vi "Get Enclosing Target Item.vi"(11 "tsRef":refnum<vi>) -> (3 "targetItem":refnum<vi>)   [LabVIEW 2020, in "NI_TargetHelper.lvlib"]
uses:
  <vilib>/TargetSupport/NI_TargetHelper/NI_TargetHelper.lvlib
  a0133eca-297a-364c-b9d3-27e53c6066f6.vi
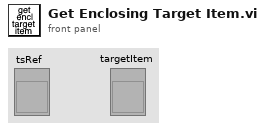
[diagram p1: front panel]
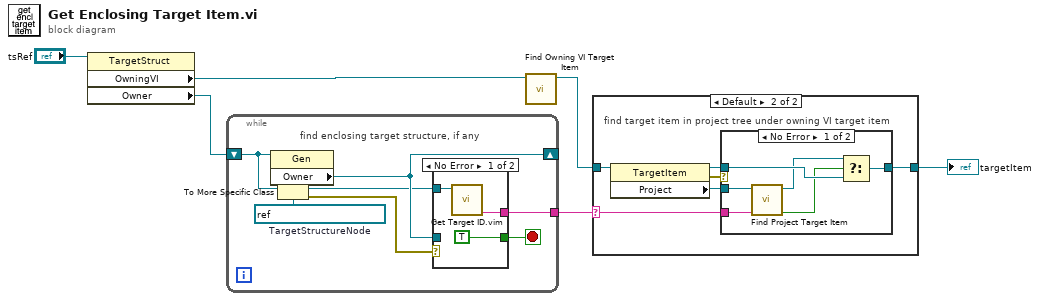
[diagram p0: block diagram]
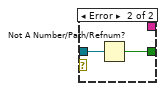
[diagram p4: hidden frame]
diagram:
  n1 = property class="TargetStruct"(reference="tsRef") -> ("OwningVI"=w3:refnum<vi>, "Owner"=w5:refnum<vi>)  [unwired: 1 in, 2 out]
  n2 = while {
    shift-right: [w9] -> _
    shift-left: w5 -> [w12]
    tunnel: [w7] -> w4
    stop <- w10 stop-if-true
    w13 = refnum<vi> refnum  # TargetStructureNode
    # "find enclosing target structure, if any"
    n3 = property class="Gen"(reference=w12) -> ("Owner"=w9:refnum<vi>)  [unwired: 1 in, 2 out]
    n4 = To More Specific Class(target class=w13, reference=w12) -> (specific class reference=w8:refnum<vi>, error out=w11:errorcluster)  [unwired: 1 in]
    n5 = case shown="No Error" w11 {
      tunnel: [TRUE w17] -> w10
      tunnel: w9 -> [_ w18]
      tunnel: w8 -> [w15 _]
      tunnel: [w14 _] -> w7
      frame No Error {
        n6 = call "Get Target ID.vim"("ref in"=w15) -> ("target ID"=w14:string)  [unwired: 9 in, 1 out]
      }
      frame Error {
        n7 = Not A Number/Path/Refnum?(number/path/refnum=w18) -> (NaN/Path/Refnum?=w17:bool)
      }
    }
  }
  n8 = call <vilib>:"Find Owning VI Target Item.vi"("viref"=w3) -> ("targetItem"=w2:refnum<vi>)  [unwired: 10 in]
  n9 = case shown="Default" w4 {
    selector: w4 -> [_ w20]
    tunnel: [w19 w23] -> w1
    tunnel: w2 -> [w19 w25]
    frame "" {
      # "no enclosing target, use owning VI target item"
    }
    frame Default {
      # "find target item in project tree under owning VI target item"
      n10 = property class="TargetItem"(reference=w25) -> (reference out=w21:refnum<vi>, error out=w22:errorcluster, "Project"=w24:refnum<vi>)  [unwired: 1 in]
      n11 = case shown="No Error" w22 {
        tunnel: w24 -> [w29 _]
        tunnel: [w31 w32] -> w23
        tunnel: w21 -> [w30 w32]
        tunnel: w20 -> [w28 _]
        frame No Error {
          n12 = call <vilib>:"Find Project Target Item.vi"("target structure name"=w28, "project"=w29) -> ("found"=w26:bool, "TargetItem Refnum"=w27:refnum<vi>)  [unwired: 8 in]
          n13 = Select(t=w27, s=w26, f=w30) -> (s? t:f=w31:refnum<vi>)
        }
        frame Error {
        }
      }
    }
  }
  "targetItem" <- w1
